vi "host_dma_read.vi"(8 "error in":errorcluster) -> (0 "error out":errorcluster, 1 "values":sgl[][](array[numeric]), 2 "indices":i16[][](array[numeric]), 3 "status":T1[](array[typedef]))   [LabVIEW 2021]
uses:
  fpga/fpga_dtype_status.ctl
  host_global_vars.vi
  <vilib>/Utility/error.llb/Error Cluster From Error Code.vi
  <vilib>/rvi/errors/niLvFpgaAdjustHostInterfaceError.vi
  <vilib>/rvi/interface/nirviMethod/nirviMethod.xnode
  FPGA Bitfiles/openlabspm_FPGATarget_fpgamain_eo-gUZR5D1g.lvbitx
  fpga/fpga_main.vi
  <vilib>/FPGAPlugInAG/PXIe-7856R/niLvFpga_ReadFifo_PXIe-7856R.vi
  <vilib>/rvi/errors/niLvFpgaMergeErrorWithErrorCode.vi
panel:
  out "Elements Remaining":u32
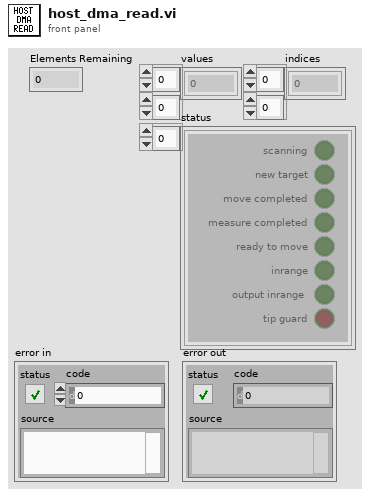
[diagram p1: front panel]
types:
  T1 = typedef "fpga_dtype_status.ctl" = cluster{"scanning":bool, "new target":bool, "move completed":bool, "measure completed":bool, "inrange":bool, "ready to move":bool, "output inrange":bool, "tip guard":bool}
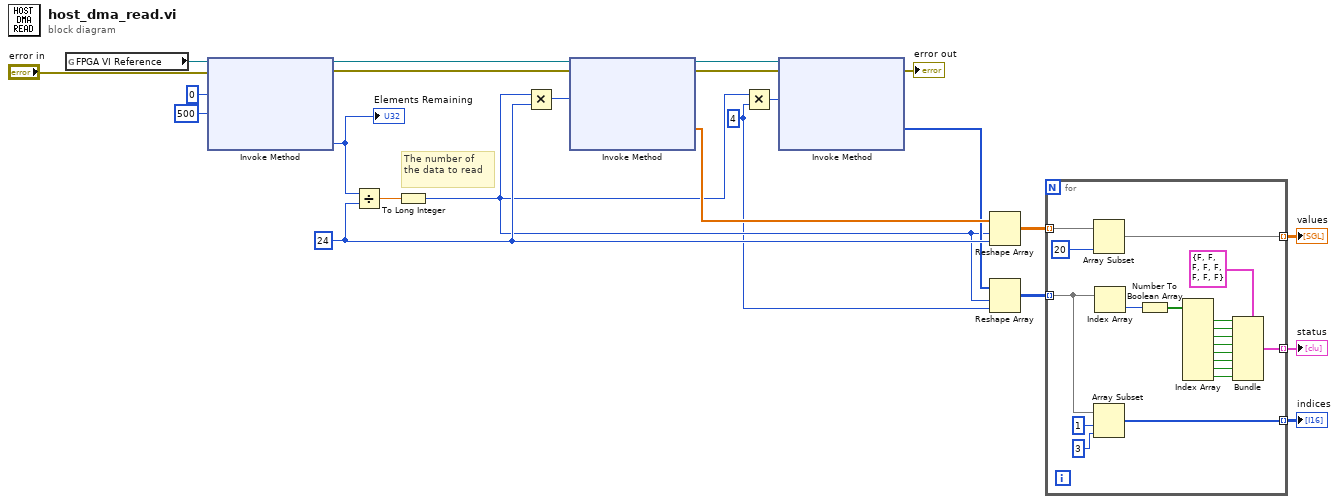
[diagram p0: block diagram]
diagram:
  w8 = 4 ("y")
  w11 = u32 24 ("y")
  # "The number of the data to read"
  n1 = global read "host_global_vars.vi" "FPGA VI Reference"() -> (w21:refnum<k20>)
  n2 = xnode "Invoke Method"("FPGA VI Reference In"=w21, "error in"="error in", "Number of Elements"=u32 0, "Timeout (ms)"=500) -> ("FPGA VI Reference Out"=w16:refnum<k20>, "error out"=w17:errorcluster, "Elements Remaining"=w20:u32)  [unwired: 1 out]
  "Elements Remaining" <- w20
  n3 = Divide(x=w20, y=w11) -> (x/y=w19:dbl)
  n4 = To Long Integer(number=w19) -> (32bit integer=w9:i32)
  n5 = Multiply(x=w9, y=w11) -> (x*y=w18:u32)
  n6 = xnode "Invoke Method"("FPGA VI Reference In"=w16, "error in"=w17, "Number of Elements"=w18) -> ("FPGA VI Reference Out"=w14:refnum<k20>, "error out"=w15:errorcluster, "Data"=w12:sgl[])  [unwired: 1 in, 1 out]
  n7 = Multiply(x=w9, y=w8) -> (x*y=w13:i32)
  n8 = xnode "Invoke Method"("FPGA VI Reference In"=w14, "error in"=w15, "Number of Elements"=w13) -> ("error out"=→"error out":errorcluster, "Data"=w10:i16[])  [unwired: 1 in, 2 out]
  n9 = Reshape Array(w12, w9, w11) -> (w7:sgl[][])
  n10 = Reshape Array(w10, w9, w8) -> (w6:i16[][])
  n11 = for {
    tunnel: w7 -> [w41] mode=indexing
    tunnel: w6 -> [w40] mode=indexing
    tunnel: [w27] -> w1 mode=indexing
    tunnel: [w26] -> w5 mode=indexing
    tunnel: [w25] -> w4 mode=indexing
    n12 = Array Subset(array=w41, length=20) -> (w27:sgl[])  [unwired: 1 in]
    n13 = Array Subset(array=w40, index=1, length=3) -> (w25:i16[])
    n14 = Index Array(array=w40) -> (element=w37:i16)  [unwired: 1 in]
    n15 = Number To Boolean Array(number=w37) -> (Boolean array=w35:bool[])
    n16 = Index Array(array=w35) -> (element #1=w34:bool, element #2=w33:bool, element #3=w32:bool, element #4=w31:bool, element #5=w30:bool, element #6=w29:bool, element #7=w28:bool, element #8=w24:bool)  [unwired: 8 in]
    n17 = Bundle(cluster=T1 {"scanning"=FALSE, "new target"=FALSE, "move completed"=FALSE, "measure completed"=FALSE, "inrange"=FALSE, "ready to move"=FALSE, "output inrange"=FALSE, "tip guard"=FALSE} ("status"), "scanning"=w34, "new target"=w33, "move completed"=w32, "measure completed"=w31, "inrange"=w30, "ready to move"=w29, "output inrange"=w28, "tip guard"=w24) -> (w26:T1)
  }
  "values" <- w1
  "status" <- w5
  "indices" <- w4
